vi "Stream to Image Files (Optimized Performance).vi"() -> ()   [LabVIEW 2023]
doc: "The Stream to Image Files (Optimized Performance) example shows how to save images to PNG files in parallel when using a ring acquisition. Images acquired from a camera are stored in a ring buffer and references to each image are pushed to a queue. Each worker loop removes a reference from the queue and saves the image to disk. When processing is complete, <B>IMAQdx Release Image</B> must be called in order to free space in the ring buffer."
uses:
  <vilib>/vision/driver/IMAQdx.llb/IMAQdx Acquisition Mode.ctl
  <vilib>/vision/Image Controls.llb/IMAQ Image.ctl
  <vilib>/vision/driver/IMAQdx.llb/IMAQdx Buffer Number Mode.ctl
  <vilib>/Utility/High Resolution Relative Seconds.vi
  <vilib>/vision/driver/NI_Vision_Acquisition_Software.lvlib
  <resource>/objmgr/imaqdx.rc
panel:
  in  "Skip Count":u32
  out "Images Saved Per Second":dbl
  in  "Stopped":bool
  out "Images Acquired Per Second":dbl
  in  "Number of Workers":u8=3 min=1 max=3
  out "Destination Folder":path
  out "Write Speed":dbl(graph) caption="Image File Write Speed"
  out "Images Behind":i32
  in  "Number of Images":i32=30
  in  "Camera Name":refnum<k21> caption="IMAQdx Session"
  in  "Stop":bool
  # "Overview: Demonstrates how to stream images to disk in parallel when using a ring acquisition.\nRequirements: Vision Acquisition Software\nInstructions:\n1. Select the Camera Name\n2. Run the VI\n3. Reduce the Number of Workers to see if the streaming of images can keep up with fewer workers.\n4. Increase the Skip Count if Images Behind is greater than 0."
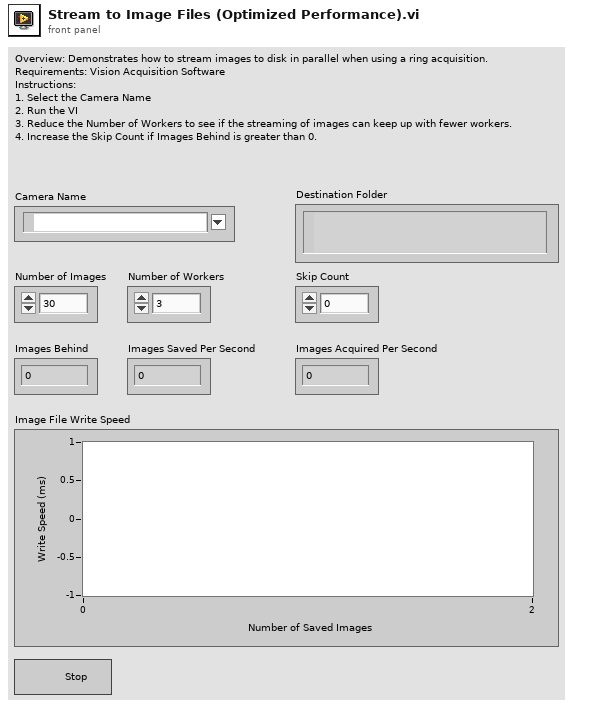
[diagram p1: front panel]
types:
  T1 = typedef "IMAQ Image.ctl" = refnum<image>
  T2 = typedef "NI_Vision_Acquisition_Software.lvlib/IMAQdx Acquisition Mode.ctl" = enum32{"One Shot", "Continuous"}
  T3 = typedef "IMAQdx.ctl" = refnum<k21>
  T4 = typedef "NI_Vision_Acquisition_Software.lvlib/IMAQdx Buffer Number Mode.ctl" = enum32{"Next", "Last", "Buffer Number", "Every", "Last New"}
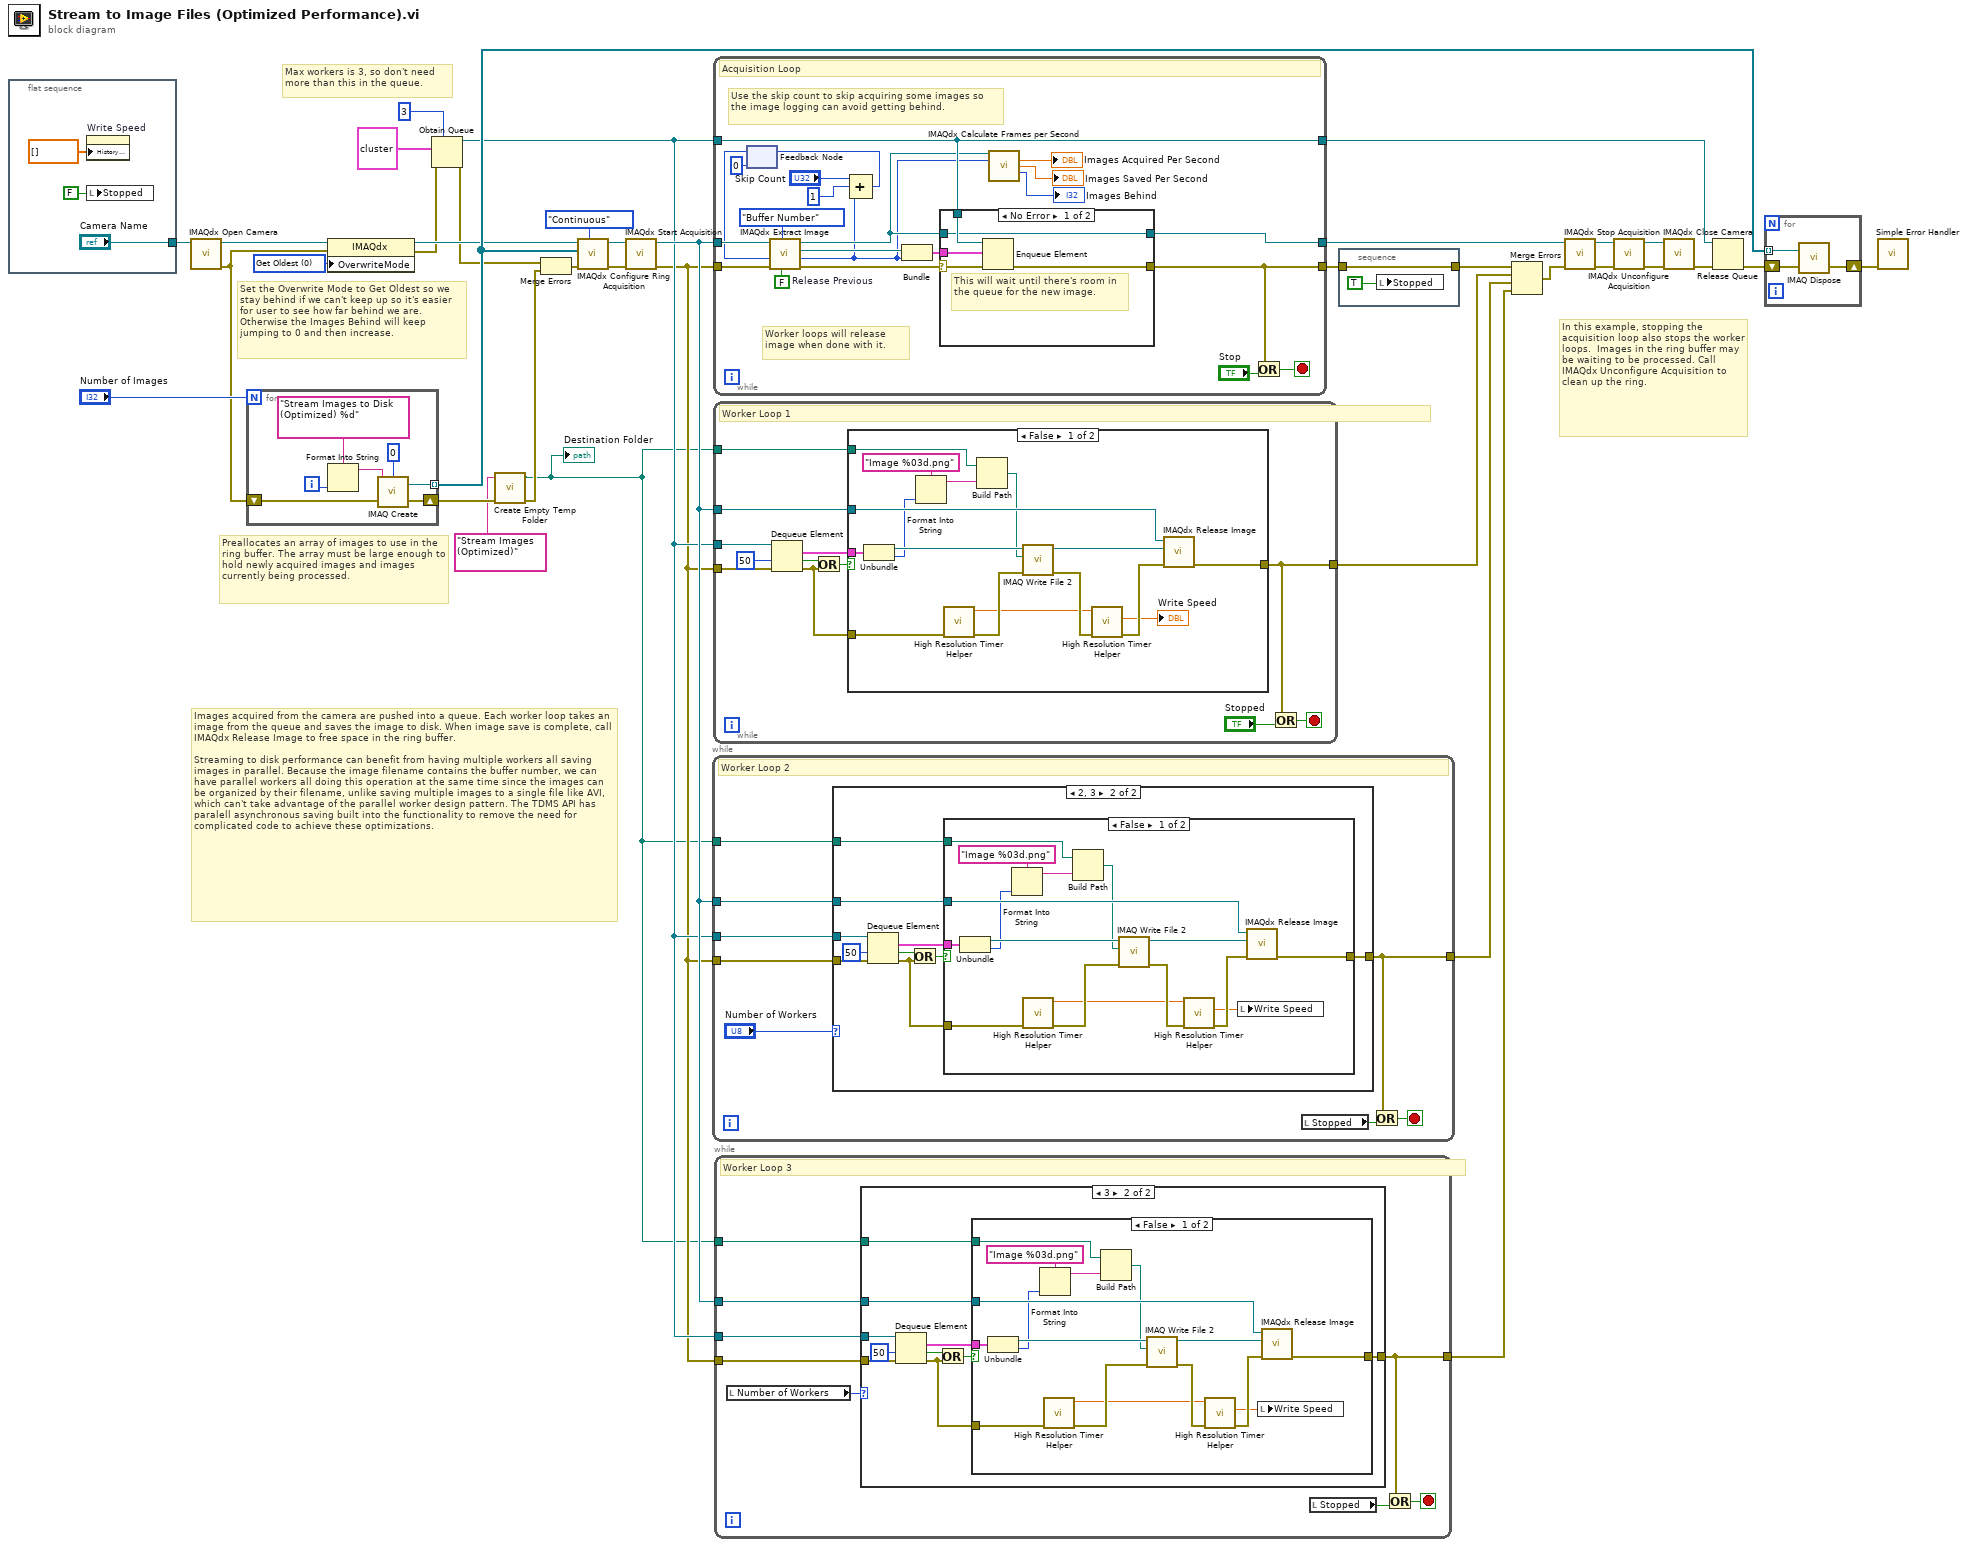
[diagram p0: block diagram]
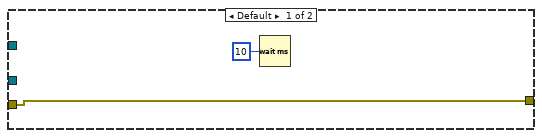
[diagram p3: hidden frame]
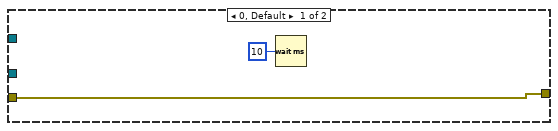
[diagram p5: hidden frame]
diagram:
  w5 = u32 0 items=["Get Oldest"=0, "Fail"=2, "Get Newest"=3] ("OverwriteMode")
  # "Set the Overwrite Mode to Get Oldest so we stay behind if we can't keep up so it's easier for user to see how far behind we are. Otherwise the Images Behind will keep jumping to 0 and then increase."
  # "Max workers is 3, so don't need more than this in the queue."
  # "In this example, stopping the acquisition loop also stops the worker loops.  Images in the ring buffer may be waiting to be processed. Call IMAQdx Unconfigure Acquisition to clean up the ring."
  # "Images acquired from the camera are pushed into a queue. Each worker loop takes an image from the queue and saves the image to disk. When image save is complete, call IMAQdx Release Image to free space in the ring buffer. \n\nStreaming to disk performance can benefit from having multiple workers all saving images in parallel. Because the image filename contains the buffer number, we can have parallel workers all doing this operation at the same time since the images can be organized by their filename, unlike saving multiple images to a single file like AVI, which can't take advantage of the parallel worker design pattern. The TDMS API has paralell asynchronous saving built into the functionality to remove the need for complicated code to achieve these optimizations."
  # "Preallocates an array of images to use in the ring buffer. The array must be large enough to hold newly acquired images and images currently being processed."
  n1 = flat-sequence {
    tunnel: ["Camera Name"] -> w36
    frame #0 {
      n2 = property on="Write Speed" class="WFChart (strict)"("History Data"=dbl[] []) -> ()  [unwired: 2 in, 2 out]
      n3 = local write "Stopped"(FALSE ("Stop")) -> ()
    }
  }
  n4 = call <vilib>:"IMAQdx Open Camera.vi"("Session In"=w36) -> ("error out"=w4:errorcluster, "Session Out"=w6:T3)  [unwired: 2 in, 7 out]
  n5 = for {
    N: "Number of Images" -> [_]
    tunnel: [w45] -> w23 mode=indexing
    shift-right: [w44] -> w11
    shift-left: w4 -> [w46]
    i -> [w43]
    n6 = Format Into String(format string="Stream Images to Disk (Optimized) %d" ("Image Name"), w43) -> (resulting string=w42:string)  [unwired: 2 in, 1 out]
    n7 = call "IMAQ Create"("Border Size"=0, "Image Name"=w42, "error in (no error)"=w46) -> ("New Image"=w45:T1, "error out"=w44:errorcluster)  [unwired: 1 in, 1 out]
  }
  n8 = property class="IMAQdx"(reference=w6, error in=w4, "OverwriteMode"=w5) -> (error out=w3:errorcluster)  [unwired: 1 out]
  n9 = Obtain Queue(max queue size (-1, unlimited)=3, element data type=cluster{"Image Out":T1, "Buffer Number Out":u32} {"Image Out"=refnum, "Buffer Number Out"=0}, error in (no error)=w3) -> (queue out=w14:refnum<queue>, error out=w2:errorcluster)  [unwired: 2 in, 1 out]
  n10 = call "Create Empty Temp Folder.vi"("error in (no error)"=w11, "Folder Name"="Stream Images (Optimized)") -> ("error out"=w10:errorcluster, "Empty Temp Folder"=w9:path)  [unwired: 8 in]
  "Destination Folder" <- w9
  n11 = Merge Errors(w2, w10) -> (w27:errorcluster)
  n12 = call <vilib>:"IMAQdx Configure Ring Acquisition.vi"("Mode"=IMAQdx_Acquisition_Mode."Continuous" ("Continuous?"), "error in"=w27, "Images"=w23, "Session In"=w6) -> ("error out"=w30:errorcluster, "Session Out"=w31:T3)  [unwired: 5 in, 1 out]
  n13 = call <vilib>:"IMAQdx Start Acquisition.vi"("error in"=w30, "Session In"=w31) -> ("error out"=w13:errorcluster, "Session Out"=w15:T3)  [unwired: 8 out]
  n14 = while {
    tunnel: w14 -> [w51]
    tunnel: w15 -> [w53]
    tunnel: w13 -> [w50]
    tunnel: w9 -> [w52]
    tunnel: [w49] -> w16
    stop <- w54 stop-if-true
    # "Worker Loop 2"
    n15 = case shown="2, 3" "Number of Workers" {
      tunnel: w53 -> [_ w61]
      tunnel: w52 -> [_ w60]
      tunnel: w51 -> [_ w59]
      tunnel: w50 -> [w56 w58]
      tunnel: [w56 w57] -> w49
      frame 0, Default {
        n16 = Wait (ms)(milliseconds to wait=u32 10) -> ()  [unwired: 1 out]
      }
      frame 2, 3 {
        n17 = Dequeue Element(queue=w59, timeout in ms (-1)=50 ("timeout in ms"), error in (no error)=w58) -> (element=w63:cluster{"Image Out":T1, "Buffer Number Out":u32}, timed out?=w65:bool, error out=w66:errorcluster)  [unwired: 1 out]
        n18 = Or(x=w65, y=w66) -> (x .or. y?=w64:bool)
        n19 = case shown="False" w64 {
          tunnel: w66 -> [w72 w83]
          tunnel: w63 -> [w82 _]
          tunnel: [w81 w83] -> w57
          tunnel: w61 -> [w80 _]
          tunnel: w60 -> [w77 _]
          frame False {
            n20 = Unbundle(w82) -> ("Image Out"=w79:T1, "Buffer Number Out"=w74:u32)
            n21 = Format Into String(format string="Image %03d.png", w74) -> (resulting string=w76:string)  [unwired: 2 in, 1 out]
            n22 = call "High Resolution Timer Helper.vi"("error in (no error)"=w72) -> ("error out"=w71:errorcluster, "Current Time"=w68:dbl)  [unwired: 8 in, 1 out]
            n23 = Build Path(base path=w77, name or relative path=w76) -> (appended path=w73:path)
            n24 = call-poly "IMAQ Write File 2"("error in (no error)"=w71, "File Path"=w73, "Image"=w79) -> ("error out"=w70:errorcluster, "Image Out (duplicate)"=w78:T1)  [unwired: 7 in]
            n25 = call "High Resolution Timer Helper.vi"("error in (no error)"=w70, "Previous Time"=w68) -> ("error out"=w69:errorcluster, "Time Difference (ms)"=w67:dbl)  [unwired: 7 in, 1 out]
            n26 = local write "Write Speed"(w67) -> ()
            n27 = call <vilib>:"IMAQdx Release Image.vi"("error in"=w69, "Image"=w78, "Session In"=w80) -> ("error out"=w81:errorcluster)  [unwired: 7 in, 1 out]
          }
          frame True {
            # "Empty queue or error.\nNothing to process."
          }
        }
      }
    }
    n28 = local read "Stopped"() -> (w47:bool)
    n29 = Or(x=w49, y=w47) -> (x .or. y?=w54:bool)
  }
  n30 = while {
    tunnel: w13 -> [w105]
    tunnel: w15 -> [w101]
    tunnel: w14 -> [w97]
    tunnel: [w96] -> w22
    tunnel: [w95] -> w19
    tunnel: [w97] -> w24
    stop <- w94 stop-if-true
    w102 = FALSE  # Release Previous
    # "Use the skip count to skip acquiring some images so the image logging can avoid getting behind."
    # "Worker loops will release image when done with it."
    # "Acquisition Loop"
    n31 = feedback #1(u32 0) -> (w92:u32)
    n32 = call <vilib>:"IMAQdx Extract Image.vi"("Release Previous (true)"=w102, "Buffer Number Mode (Next)"=IMAQdx_Buffer_Number_Mode."Buffer Number" ("Buffer Number Mode"), "error in"=w105, "Buffer Number In"=w92, "Session In"=w101) -> ("error out"=w100:errorcluster, "Buffer Number Out"=w84:u32, "Image Out"=w99:T1, "Session Out"=w85:T3)  [unwired: 3 in]
    n33 = Compound Arithmetic op=ADD("Skip Count", u32 1 ("value"), w84) -> (w93:u32)
    n34 = feedback-in #1(w93) -> ()
    n35 = Bundle("Image Out"=w99, "Buffer Number Out"=w84) -> (w98:cluster{"Image Out":T1, "Buffer Number Out":u32})  [unwired: 1 in]
    n36 = case shown="No Error" w100 {
      selector: w100 -> [w110 w111]
      tunnel: [w106 w112] -> w96
      tunnel: w85 -> [w106 w112]
      tunnel: w98 -> [w109 _]
      tunnel: w97 -> [w108 _]
      tunnel: [w107 w111] -> w95
      frame No Error {
        # "This will wait until there's room in the queue for the new image."
        n37 = Enqueue Element(queue=w108, element=w109, error in (no error)=w110) -> (error out=w107:errorcluster)  [unwired: 1 in, 2 out]
      }
      frame Error {
      }
    }
    n38 = call <vilib>:"IMAQdx Calculate Frames per Second.vi"("Session In"=w85, "Buffer Number"=w84) -> ("Acquired Frames per Second"=→"Images Acquired Per Second":dbl, "Processed Frames per Second"=→"Images Saved Per Second":dbl, "Images Behind"=→"Images Behind":i32)  [unwired: 7 in, 4 out]
    n39 = Or(x=w95, y="Stop") -> (x .or. y?=w94:bool)
  }
  n40 = while {
    tunnel: w14 -> [w116]
    tunnel: w15 -> [w118]
    tunnel: w13 -> [w115]
    tunnel: w9 -> [w117]
    tunnel: [w114] -> w17
    stop <- w124 stop-if-true
    # "Worker Loop 1"
    n41 = Dequeue Element(queue=w116, timeout in ms (-1)=50 ("timeout in ms"), error in (no error)=w115) -> (element=w120:cluster{"Image Out":T1, "Buffer Number Out":u32}, timed out?=w122:bool, error out=w123:errorcluster)  [unwired: 1 out]
    n42 = Or(x=w122, y=w123) -> (x .or. y?=w121:bool)
    n43 = case shown="False" w121 {
      tunnel: w123 -> [w130 w141]
      tunnel: w120 -> [w140 _]
      tunnel: [w139 w141] -> w114
      tunnel: w118 -> [w138 _]
      tunnel: w117 -> [w135 _]
      frame False {
        n44 = Unbundle(w140) -> ("Image Out"=w137:T1, "Buffer Number Out"=w132:u32)
        n45 = Format Into String(format string="Image %03d.png", w132) -> (resulting string=w134:string)  [unwired: 2 in, 1 out]
        n46 = call "High Resolution Timer Helper.vi"("error in (no error)"=w130) -> ("error out"=w129:errorcluster, "Current Time"=w127:dbl)  [unwired: 8 in, 1 out]
        n47 = Build Path(base path=w135, name or relative path=w134) -> (appended path=w131:path)
        n48 = call-poly "IMAQ Write File 2"("error in (no error)"=w129, "File Path"=w131, "Image"=w137) -> ("error out"=w128:errorcluster, "Image Out (duplicate)"=w136:T1)  [unwired: 7 in]
        n49 = call "High Resolution Timer Helper.vi"("error in (no error)"=w128, "Previous Time"=w127) -> ("error out"=w126:errorcluster, "Time Difference (ms)"=→"Write Speed":dbl)  [unwired: 7 in, 1 out]
        n50 = call <vilib>:"IMAQdx Release Image.vi"("error in"=w126, "Image"=w136, "Session In"=w138) -> ("error out"=w139:errorcluster)  [unwired: 7 in, 1 out]
      }
      frame True {
        # "Empty queue or error.\nNothing to process."
      }
    }
    n51 = Or(x=w114, y="Stopped") -> (x .or. y?=w124:bool)
  }
  n52 = while {
    tunnel: w14 -> [w146]
    tunnel: w15 -> [w148]
    tunnel: w13 -> [w145]
    tunnel: w9 -> [w147]
    tunnel: [w144] -> w12
    stop <- w149 stop-if-true
    # "Worker Loop 3"
    n53 = local read "Number of Workers"() -> (w143:u8)
    n54 = case shown="3" w143 {
      tunnel: w148 -> [_ w156]
      tunnel: w147 -> [_ w155]
      tunnel: w146 -> [_ w154]
      tunnel: w145 -> [w151 w153]
      tunnel: [w151 w152] -> w144
      frame Default {
        n55 = Wait (ms)(milliseconds to wait=u32 10) -> ()  [unwired: 1 out]
      }
      frame 3 {
        n56 = Dequeue Element(queue=w154, timeout in ms (-1)=50 ("timeout in ms"), error in (no error)=w153) -> (element=w158:cluster{"Image Out":T1, "Buffer Number Out":u32}, timed out?=w160:bool, error out=w161:errorcluster)  [unwired: 1 out]
        n57 = Or(x=w160, y=w161) -> (x .or. y?=w159:bool)
        n58 = case shown="False" w159 {
          tunnel: w161 -> [w167 w178]
          tunnel: w158 -> [w177 _]
          tunnel: [w176 w178] -> w152
          tunnel: w156 -> [w175 _]
          tunnel: w155 -> [w172 _]
          frame False {
            n59 = Unbundle(w177) -> ("Image Out"=w174:T1, "Buffer Number Out"=w169:u32)
            n60 = Format Into String(format string="Image %03d.png", w169) -> (resulting string=w171:string)  [unwired: 2 in, 1 out]
            n61 = call "High Resolution Timer Helper.vi"("error in (no error)"=w167) -> ("error out"=w166:errorcluster, "Current Time"=w164:dbl)  [unwired: 8 in, 1 out]
            n62 = Build Path(base path=w172, name or relative path=w171) -> (appended path=w168:path)
            n63 = call-poly "IMAQ Write File 2"("error in (no error)"=w166, "File Path"=w168, "Image"=w174) -> ("error out"=w165:errorcluster, "Image Out (duplicate)"=w173:T1)  [unwired: 7 in]
            n64 = call "High Resolution Timer Helper.vi"("error in (no error)"=w165, "Previous Time"=w164) -> ("error out"=w163:errorcluster, "Time Difference (ms)"=w162:dbl)  [unwired: 7 in, 1 out]
            n65 = local write "Write Speed"(w162) -> ()
            n66 = call <vilib>:"IMAQdx Release Image.vi"("error in"=w163, "Image"=w173, "Session In"=w175) -> ("error out"=w176:errorcluster)  [unwired: 7 in, 1 out]
          }
          frame True {
            # "Empty queue or error.\nNothing to process."
          }
        }
      }
    }
    n67 = local read "Stopped"() -> (w142:bool)
    n68 = Or(x=w144, y=w142) -> (x .or. y?=w149:bool)
  }
  n69 = stacked-sequence {
    tunnel: [w180] -> w18
    tunnel: w19 -> [w180]
    frame #0 {
      n70 = local write "Stopped"(TRUE ("Stop")) -> ()
    }
  }
  n71 = Merge Errors(w18, w17, w16, w12) -> (w26:errorcluster)
  n72 = call <vilib>:"IMAQdx Stop Acquisition.vi"("error in"=w26, "Session In"=w22) -> ("error out"=w32:errorcluster, "Session Out"=w33:T3)  [unwired: 8 out]
  n73 = call <vilib>:"IMAQdx Unconfigure Acquisition.vi"("error in"=w32, "Session In"=w33) -> ("error out"=w35:errorcluster, "Session Out"=w34:T3)  [unwired: 8 out]
  n74 = call <vilib>:"IMAQdx Close Camera.vi"("error in"=w35, "Session In"=w34) -> ("error out"=w21:errorcluster)  [unwired: 9 out]
  n75 = Release Queue(queue=w24, error in (no error)=w21) -> (error out=w20:errorcluster)  [unwired: 1 in, 2 out]
  n76 = for {
    shift-right: [w182] -> w1
    shift-left: w20 -> [w183]
    tunnel: w23 -> [w181] mode=indexing
    n77 = call "IMAQ Dispose"("Image"=w181, "error in (no error)"=w183) -> ("error out"=w182:errorcluster)  [unwired: 4 in]
  }
  n78 = call <vilib>:"Simple Error Handler.vi"("error in (no error)"=w1) -> ()  [unwired: 4 in, 5 out]
